vi "Simplified UART loop.vi"() -> ()   [LabVIEW 2017]
uses:
  <vilib>/myRIO/Instrument Drivers/Onboard IO/UART/typedef/VISA Configuration.ctl
  <vilib>/myRIO/Instrument Drivers/Onboard IO/UART/UART.lvlib
panel:
  out "error?":bool
  in  "stop":bool
  out "read buffer":string
  in  "Read mode":enum16{"Read all", "Get latest value"}(ring)=enum."Get latest value"
  in  "VISA resource name in":refnum<visa-resource-name>="ASRL1::INSTR"
  out "timeout (10sec)":u32
  in  "input cluster":T1={"baud rate (9600)"=115200, "data bits (8)"=8, "parity (0:none)"=enum."None", "stop bits (10: 1 bit)"=10, "flow control (0:none)"=0, "termination char\n(0xA = '\\n' = LF) "=10, "Enable Termination\nChar (T)"=TRUE, "timeout (10sec)"=1000} {"termination char\n(0xA = '\\n' = LF)" format="%.0x"; "flow control (0:none)" items=["None", "XON/XOFF", "RTS/CTS", "XON/XOFF & RTS/CTS", "DTR/DSR", "XON/XOFF & DTR/DSR"]; "stop bits (10: 1 bit)" items=["1.0"=10, "1.5"=15, "2.0"=20]; "data bits (8)" min=5 max=8 step=1}
  out "error out":errorcluster
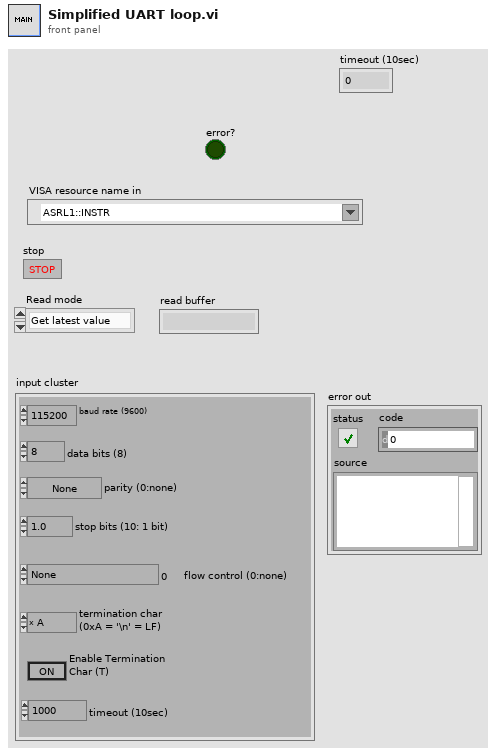
[diagram p1: front panel]
types:
  T1 = typedef "UART.lvlib/VISA Configuration.ctl" = cluster{"baud rate (9600)":u32, "data bits (8)":u16, "parity (0:none)":enum16{"None", "Odd", "Even", "Mark", "Space"}, "stop bits (10: 1 bit)":u16, "flow control (0:none)":u16, "termination char\n(0xA = '\\n' = LF) ":u8, "Enable Termination\nChar (T)":bool, "timeout (10sec)":u32}
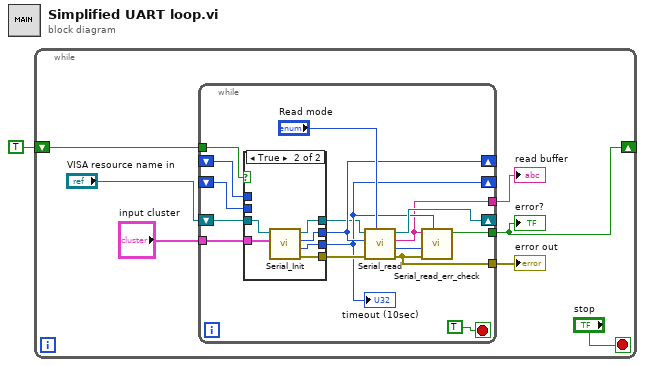
[diagram p0: block diagram]
diagram:
  n1 = while {
    shift-right: [w2] -> _
    shift-left: TRUE ("error?") -> [w6]
    stop <- "stop" stop-if-true
    n2 = while {
      shift-right: [w23] -> _
      shift-left: "VISA resource name in" -> [w15]
      shift-right: [w20] -> _
      shift-left: _ -> [w19]
      shift-right: [w18] -> _
      shift-left: _ -> [w17]
      tunnel: [w13] -> w2
      tunnel: w6 -> [w12]
      tunnel: "input cluster" -> [w11]
      tunnel: [w10] -> w4
      tunnel: [w9] -> w3
      stop <- TRUE stop-if-true
      n3 = case shown="True" w12 {
        tunnel: [_ w33] -> w21
        tunnel: [w26 w32] -> w18
        tunnel: [w27 w31] -> w20
        tunnel: w19 -> [w27 _]
        tunnel: w17 -> [w26 _]
        tunnel: [w25 w30] -> w16
        tunnel: w15 -> [w25 w29]
        tunnel: w11 -> [_ w28]
        frame False {
        }
        frame True {
          n4 = call "Serial_Init.vi"("input cluster"=w28, "VISA Refnum in"=w29) -> ("error out"=w33:errorcluster, "timeout (10sec)"=w32:u32, "Bytes at Port"=w31:u32, "VISA Refnum out"=w30:refnum<visa-resource-name>)  [unwired: 6 in]
        }
      }
      "timeout (10sec)" <- w18
      n5 = call "Serial_read.vi"("Read mode"="Read mode", "error in (no error)"=w21, "Bytes at Port"=w20, "VISA Refnum in"=w16) -> ("error out"=w10:errorcluster, "dt"=w22:u32, "read buffer"=w9:string, "VISA resource name out"=w23:refnum<visa-resource-name>)  [unwired: 4 in]
      n6 = call "Serial_read_err_check.vi"("timeout"=w18, "error in (no error)"=w10, "dt"=w22, "read buffer"=w9) -> ("error?"=w13:bool)  [unwired: 7 in]
    }
    "error out" <- w4
    "read buffer" <- w3
    "error?" <- w2
  }
